vi "GetStatusInformation.vi"(9 "HighSpeedEServer":refnum<k24>, 11 "error in (no error)":errorcluster) -> (1 "Status":T1, 3 "error out":errorcluster)   [LabVIEW 2022 SP3, in "UnderAutomation.Yaskawa.lvlib"]
uses:
  UnderAutomation.Yaskawa.lvlib
  C:/Users/fg/Documents/Yaskawa.vi/LabVIEW_2024/UnderAutomation.Yaskawa/lib/UnderAutomation.Yaskawa.dll
  LabVIEW_2024/UnderAutomation.Yaskawa/lib/UnderAutomation.Yaskawa.dll
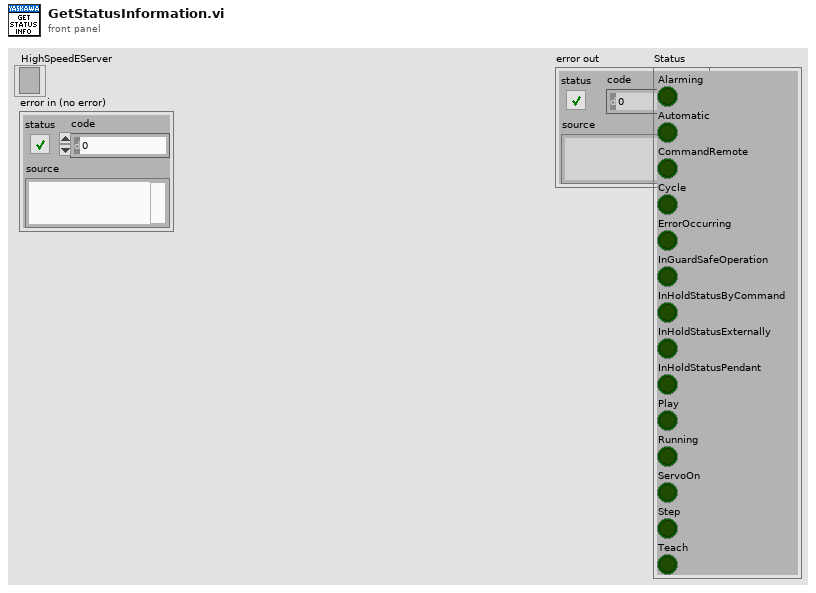
[diagram p1: front panel]
types:
  T1 = cluster{"Alarming":bool, "Automatic":bool, "CommandRemote":bool, "Cycle":bool, "ErrorOccurring":bool, "InGuardSafeOperation":bool, "InHoldStatusByCommand":bool, "InHoldStatusExternally":bool, "InHoldStatusPendant":bool, "Play":bool, "Running":bool, "ServoOn":bool, "Step":bool, "Teach":bool}
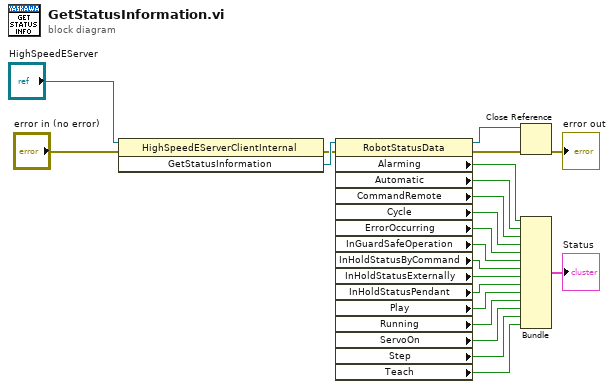
[diagram p0: block diagram]
diagram:
  n1 = invoke class="HighSpeedEServerClientInternal" method="GetStatusInformation"(reference="HighSpeedEServer", error in="error in (no error)") -> (error out=w19:errorcluster, "GetStatusInformation"=w20:refnum<k24>)  [unwired: 1 in, 1 out]
  n2 = property class="RobotStatusData"(reference=w20, error in=w19) -> (reference out=w1:refnum<k24>, error out=w3:errorcluster, "Alarming"=w18:bool, "Automatic"=w17:bool, "CommandRemote"=w16:bool, "Cycle"=w15:bool, "ErrorOccurring"=w14:bool, "InGuardSafeOperation"=w13:bool, "InHoldStatusByCommand"=w12:bool, "InHoldStatusExternally"=w11:bool, "InHoldStatusPendant"=w10:bool, "Play"=w9:bool, "Running"=w8:bool, "ServoOn"=w7:bool, "Step"=w6:bool, "Teach"=w5:bool)
  n3 = Close Reference(reference=w1, error in (no error)=w3) -> (error out=→"error out":errorcluster)
  n4 = Bundle("Alarming"=w18, "Automatic"=w17, "CommandRemote"=w16, "Cycle"=w15, "ErrorOccurring"=w14, "InGuardSafeOperation"=w13, "InHoldStatusByCommand"=w12, "InHoldStatusExternally"=w11, "InHoldStatusPendant"=w10, "Play"=w9, "Running"=w8, "ServoOn"=w7, "Step"=w6, "Teach"=w5) -> (→"Status":T1)  [unwired: 1 in]
